vi "Error Handlers.vi"   [LabVIEW 2020, in "NI_AAL_Filter.lvlib"]
uses:
  <vilib>/Analysis/NI_AAL_Filter.lvlib
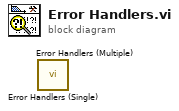
[diagram p0: block diagram]
diagram:
  n1 = call <vilib>:"Error Handlers (Single).vi"() -> ()  [unwired: 11 in, 1 out]
  n2 = call <vilib>:"Error Handlers (Multiple).vi"() -> ()  [unwired: 11 in, 1 out]
